vi "add.vi"(1 "Slide":dbl, 2 "Numeric 2":dbl) -> (0 "Numeric":dbl)   [LabVIEW 2010]
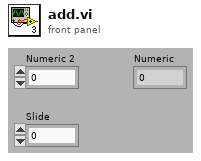
[diagram p1: front panel]
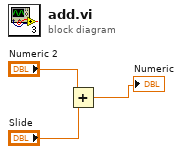
[diagram p0: block diagram]
diagram:
  n1 = Add(x="Numeric 2", y="Slide") -> (x+y=→"Numeric":dbl)
